vi "RealSense_HelloWorld_Depth_and_Color.vi"() -> ()   [LabVIEW 2023]
doc: "Simple Demo showing how to connect a RealSense Camera to stream COLOR and DEPTH from the stereo camera of a D4xx series camera."
panel:
  out "Output stream format":T1={"width"=1280, "height"=720, "fps"=30, "Profile"=605382696, "ppx"=634.5728, "ppy"=370.69974, "fx"=952.6064, "fy"=952.6064, "model"=4}
  in  "Color Presets":T2(ring)=enum."D435"
  in  "Depth Presets":T3(ring)=enum."Original"
  in  "laser on/off":bool=TRUE
  in  "autoexposure":bool=TRUE
  in  "Laser power, mW":sgl=150.0
  in  "Gain(16-248)":sgl=64.0
  in  "Exposure,us":sgl=156.0
  out "Depth map":sgl[][](graph)
  out "RGB image":picture
  out "iteration":i32=22
  in  "stop":bool=TRUE
  out "release frame error":string="No Error"
  out "Capture1 Error":string="No Error"
  out "Config error":string="No Error\rNo Error"
  out "init results":T4={"camera name"="Intel RealSense 415", "camera S/N"="725112060291", "F/W"="05.08.08.00", "Sensor name"="Stereo Module", "api_version"=20801, "rscontext"=606847696, "device_list"=597043920, "device count"=2, "Dev out"=606875504, "sensor_list"=605604656, "sensor count"=2, "Sensor out"=601640400}
  out "init error":string="No Error\rNo Error\rNo Error\rNo Error\rNo Error\rNo Error\rNo Error\rNo Error\rNo Error\rNo Error\rNo Error"
  out "Close Error":string="No Error\rNo Error\rNo Error\rNo Error"
  out "Start Error":string="No Error\rNo Error\rNo Error"
  out "Capture2 error":string="No Error"
  in  "Select Resolution":u16(ring)=15 items=["424 x 240 @6fps", "424 x 240 @15fps", "424 x 240 @30fps", "424 x 240 @60fps", "424 x 240 @90fps", "480 x 270 @6fps", "480 x 270 @15fps", "480 x 270 @30fps", "480 x 270 @60fps", "480 x 270 @90fps", "640 x 360 @6fps", "640 x 360 @15fps", "640 x 360 @30fps", "640 x 360 @60fps", "640 x 360 @90fps", "640 x 480 @6fps", "640 x 480 @15fps", "640 x 480 @30fps", "640 x 480 @60fps", "640 x 480 @90fps", "848 x 480 @6fps", "848 x 480 @15fps", "848 x 480 @30fps", "848 x 480 @60fps", "848 x 480 @90fps", "1280 x 720 @6fps", "1280 x 720 @15fps", "1280 x 720 @30fps"]
  # "RealSense Hello World: Color + Depth"
  # "This demo shows how to connect a RealSense D4xx Stereo Depth Camera, and stream the COLOR (left) and a DEPTH MAP."
  # "COLOR"
  # "DEPTH MAP"
  # "Note; When you change Depth Preset you need to stop and restart for the HDAD settings to take effect.\n\nTry the Color preset called \"Remove IR2\". It will remove the laser projector from the RGB 1280x720 image."
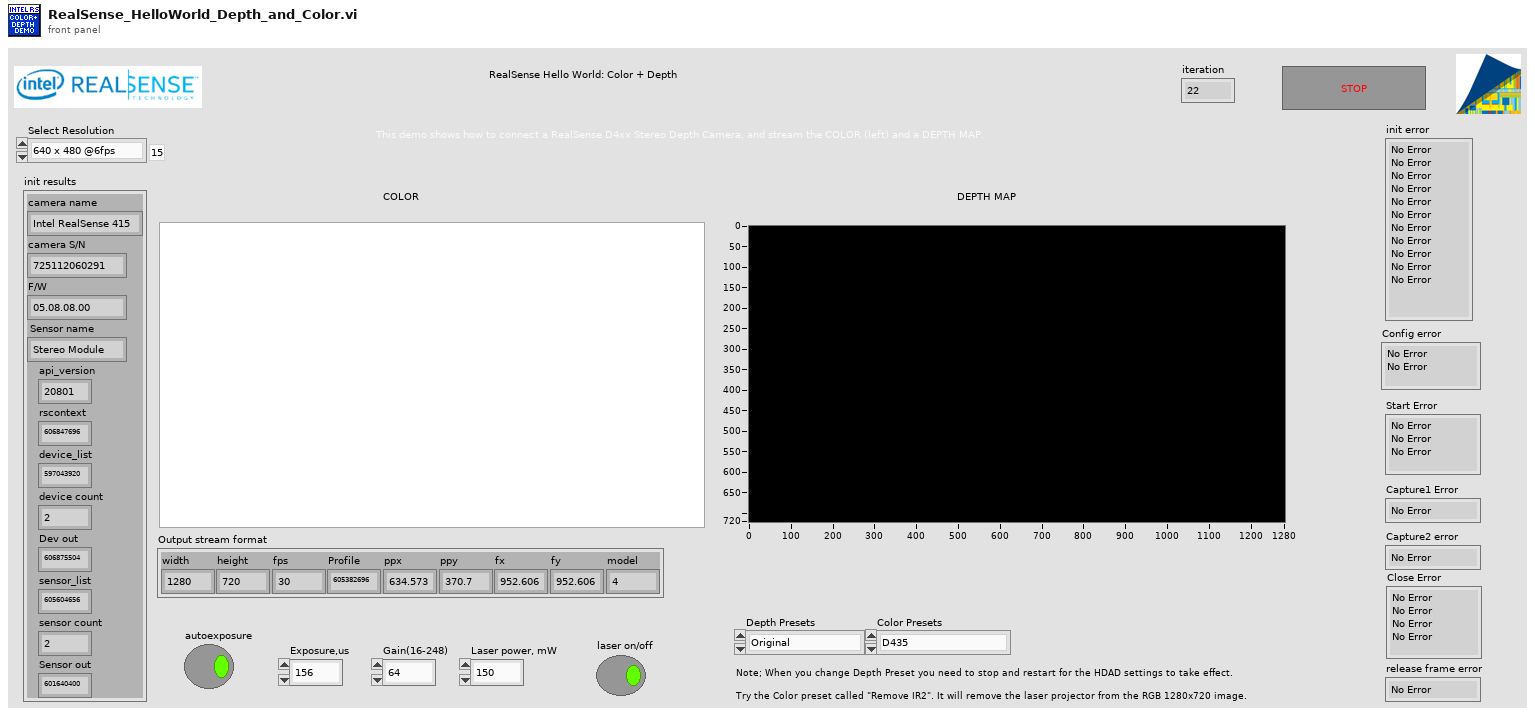
[diagram p1: front panel]
types:
  T1 = cluster{"width":i32, "height":i32, "fps":i32, "Profile":u64, "ppx":sgl, "ppy":sgl, "fx":sgl, "fy":sgl, "model":u32}
  T2 = enum16{"Custom", "RS400 (DS5p)", "RS400 (DS5p) 2", "RS400 (DS5p) 3", "RS400 (DS5p) 4", "RS400 (DS5p) 5", "RS410 (DS5a)", "RS410 (DS5a) 2", "DS410 (DS5a) 3", "DS410 (DS5a) 4", "DS410+IR", "DS5LR", "DS5LR-2", "DS5LR no pattern", "RS410 Remove IR", "RS410 Remove IR 2", "DS5micro", "D435"}
  T3 = enum16{"Custom", "Original", "New Depth 1", "New Depth 2", "Depth Active 1", "Active 3D Scan", "Active Short A", "Active Short C", "Face", "Face2", "Best Box", "High Density", "Medium Density", "High Accuracy", "Hand", "Short Range", "Flat wall", "Load .JSON", "Load .JSON2"}
  T4 = cluster{"camera name":string, "camera S/N":string, "F/W":string, "Sensor name":string, "api_version":i32, "rscontext":u64, "device_list":u64, "device count":i32, "Dev out":u64, "sensor_list":u64, "sensor count":i32, "Sensor out":u64}
  T5 = enum16{"Depth", "Color (ext.)", "Color (left) ", "IR Left", "IR Right", "IR Left (Y16)", "IR Right (Y16)"}
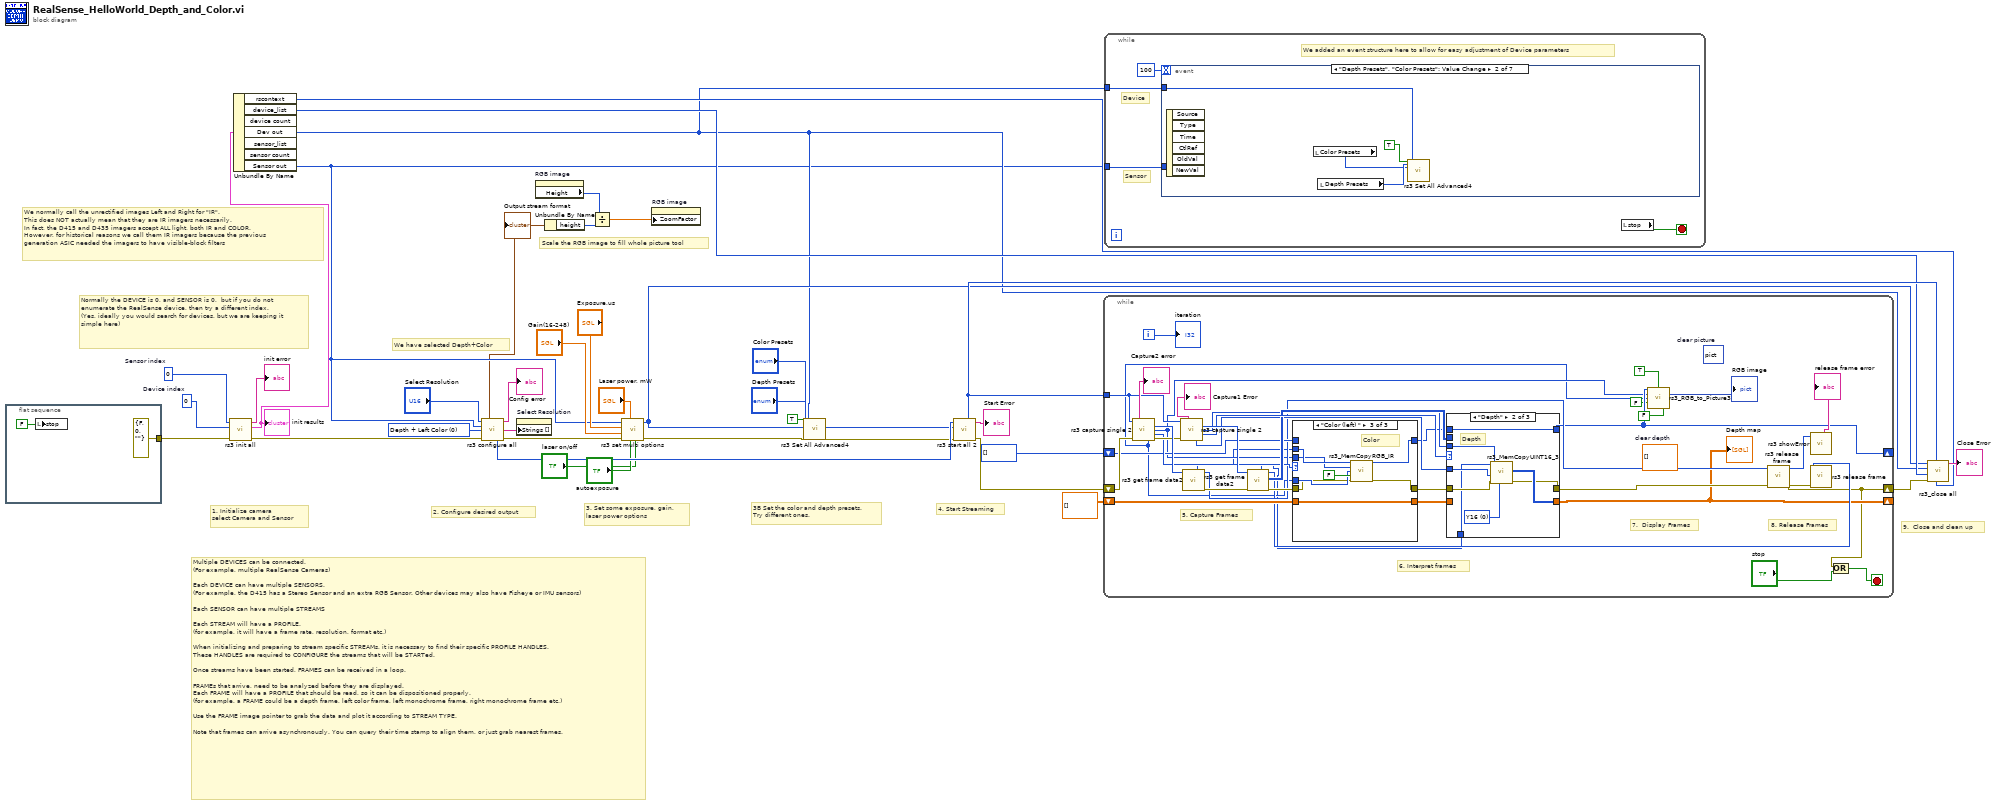
[diagram p0: block diagram]
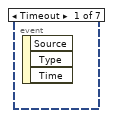
[diagram p2: hidden frame]
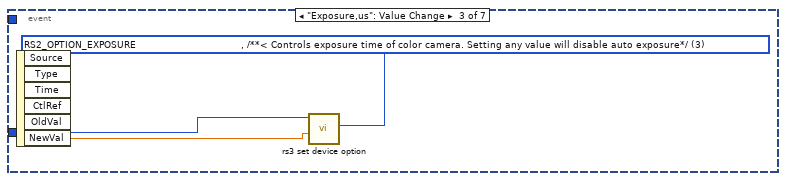
[diagram p3: hidden frame]
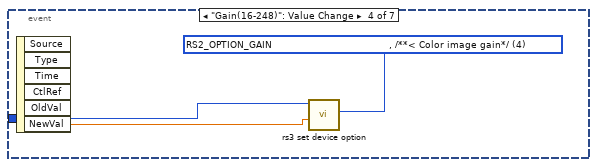
[diagram p4: hidden frame]
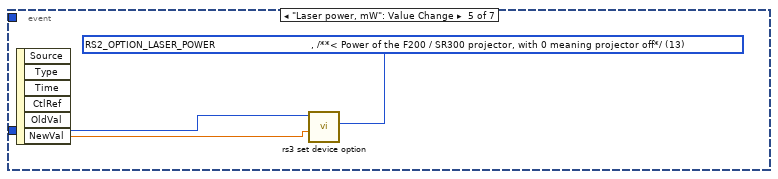
[diagram p5: hidden frame]
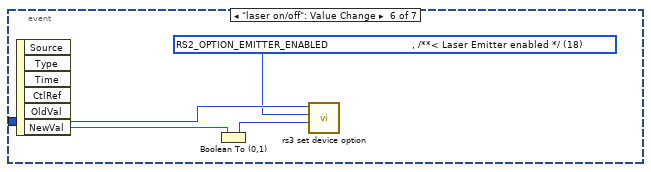
[diagram p6: hidden frame]
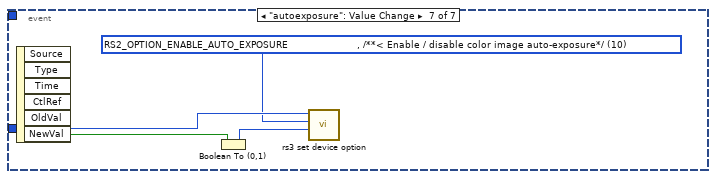
[diagram p7: hidden frame]
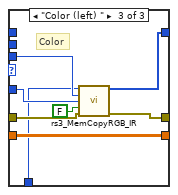
[diagram p9: hidden frame]
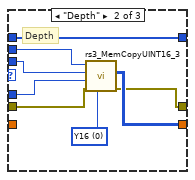
[diagram p11: hidden frame]
diagram:
  w38 = 0  # Device index
  w37 = 0  # Sensor index
  w21 = u16 0 items=["Depth + Left Color", "Unrectified L + R", "Rectified L + R"] ("Stream selection")
  # "Scale the RGB image to fill whole picture tool"
  # "3B Set the color and depth presets.\nTry different ones."
  # "We normally call the unrectified images Left and Right for \"IR\". \nThis does NOT actually mean that they are IR imagers necessarily. \nIn fact, the D415 and D435 imagers accept ALL light, both IR and COLOR.\nHowever, for historical reasons we call them IR imagers because the previous generation ASIC needed the imagers to have visible-block filters"
  # "We have selected Depth+Color"
  # "Normally the DEVICE is 0, and SENSOR is 0,  but if you do not enumerate the RealSense device, then try a different index.\n(Yes, ideally you would search for devices, but we are keeping it simple here)"
  # "Multiple DEVICES can be connected. \n(For example, multiple RealSense Cameras)\n\nEach DEVICE can have multiple SENSORS. \n(For example, the D415 has a Stereo Sensor and an extra RGB Sensor. Other devices may also have Fisheye or IMU sensors) \n\nEach SENSOR can have multiple STREAMS\n\nEach STREAM will have a PROFILE. \n(for example, it will have a frame rate, resolution, format etc.)\n\nWhen initializing and preparing to stream specific STREAMs, it is necessary to find their specific PROFILE HANDLES.\nThese HANDLES are required to CONFIGURE the streams that will be STARTed. \n\nOnce streams have been started, FRAMES can be received in a loop. \n \nFRAMEs that arrive, need to be analyzed before they are displayed. \nEach FRAME will have a PROFILE that should be read, so it can be dispositioned properly.\n(for example, a FRAME could be a depth frame, left color frame, left monochrome frame, right monochrome frame etc.)\n\nUse the FRAME image pointer to grab the data and plot it according to STREAM TYPE.\n\nNote that frames can arrive asynchronously. You can query their time stamp to align them, or just grab nearest frames."
  # "9.  Close and clean up"
  # "4. Start Streaming"
  # "3. Set some exposure, gain, \nlaser power options"
  # "2. Configure desired output"
  # "1. Initialize camera\nselect Camera and Sensor"
  n1 = flat-sequence {
    tunnel: [errorcluster {"status"=FALSE, "code"=0, "source"=""} ("error in")] -> w22
    frame #0 {
      n2 = local write "stop"(FALSE ("stop")) -> ()
    }
  }
  n3 = call "rs3 init all.vi"("error in"=w22, "Select Device"=w38, "Select Sensor"=w37) -> ("error out"=w36:errorcluster, "init results"=w29:T4, "init error"=→"init error":string)  [unwired: 2 in, 4 out]
  "init results" <- w29
  n4 = Unbundle By Name(w29) -> ("rscontext"=w27:u64, "device_list"=w28:u64, "Dev out"=w7:u64, "Sensor out"=w6:u64)  [unwired: 3 out]
  n5 = call "rs3 configure all.vi"("Select Resolution"="Select Resolution", "Sensor in"=w6, "Stream selection"=w21, "error in (no error)"=w36) -> ("Output stream L"=w4:T1, "config error"=→"Config error":string, "Output stream"=w23:string[], "Stream Profile Handles"=w35:u64[], "error out"=w20:errorcluster)  [unwired: 2 in, 5 out]
  "Output stream format" <- w4
  n6 = property on="Select Resolution" class="Ring (strict)"("Strings []"=w23) -> ()  [unwired: 2 in, 2 out]
  n7 = property on="RGB image" class="Pict"() -> ("Height"=w1:u32)  [unwired: 2 in, 2 out]
  n8 = Unbundle By Name(w4) -> ("height"=w2:i32)
  n9 = Divide(x=w1, y=w2) -> (x/y=w3:dbl)
  n10 = call "rs3 set multi options.vi"("laser on/off"="laser on/off", "autoexposure"="autoexposure", "Laser power, mW (0-360)"="Laser power, mW", "error in (no error)"=w20, "Gain(16-248)"="Gain(16-248)", "Exposure, us"="Exposure,us", "Sensor in"=w6) -> ("error out"=w12:errorcluster, "Sensor out"=w19:u64)  [unwired: 2 in, 1 out]
  n11 = property on="RGB image" class="Pict"("ZoomFactor"=w3) -> ()  [unwired: 2 in, 2 out]
  n12 = call "rs3 Set All Advanced4.vi"("Set Color Corr"=TRUE, "Depth Presets"="Depth Presets", "Color Presets"="Color Presets", "error in (no error)"=w12, "device in"=w7) -> ("error out"=w11:errorcluster)  [unwired: 20 in, 2 out]
  n13 = call "rs3 start all 2.vi"("error in (no error)"=w11, "Sensor in"=w19, "Stream profile array"=w35) -> ("error out"=w24:errorcluster, "Config Error"=→"Start Error":string, "queue out"=w34:u64)  [unwired: 5 in, 1 out]
  n14 = while {
    tunnel: w34 -> [w71]
    shift-right: [w46] -> _
    shift-left: sgl[][] [] ("2D Array Output") -> [w59]
    shift-right: [w53] -> _
    shift-left: u8[] [] ("Output Array") -> [w57]
    shift-right: [w41] -> w33
    shift-left: w24 -> [w79]
    i -> [w78]
    stop <- w42 stop-if-true
    (unwired) picture bytes[33]  # clear picture
    (unwired) sgl[][] []  # clear depth
    # "8. Release Frames"
    # "7.  Display Frames"
    # "6. Interpret frames"
    # "5. Capture Frames"
    n15 = call "rs3 capture single 2.vi"("queue in"=w71, "error in (no error)"=w79) -> ("Capture Error"=→"Capture2 error":string, "frame out"=w77:u64, "width"=w51:i32, "Stream type"=w60:T5, "height"=w50:i32, "error out"=w72:errorcluster)  [unwired: 3 in, 5 out]
    n16 = call "rs3 capture single 2.vi"("queue in"=w71, "error in (no error)"=w72) -> ("Capture Error"=→"Capture1 Error":string, "frame out"=w69:u64, "width"=w62:i32, "Stream type"=w64:T5, "height"=w61:i32)  [unwired: 3 in, 6 out]
    n17 = call "rs3 get frame data2.vi"("device in"=w77) -> ("error out"=w75:errorcluster, "device out"=w55:u64, "image pointer out"=w45:u64)  [unwired: 6 in, 2 out]
    n18 = call "rs3 get frame data2.vi"("error in (no error)"=w75, "device in"=w69) -> ("error out"=w74:errorcluster, "2D Depth Output"=w63:u16[][], "device out"=w54:u64, "image pointer out"=w44:u64)  [unwired: 5 in, 1 out]
    n19 = case shown="\"Color (left) \"" w60 {
      tunnel: [w101 w106 w113] -> w66
      tunnel: w45 -> [_ w102 w116]
      tunnel: w51 -> [_ w104 w115]
      tunnel: w50 -> [_ w103 w114]
      tunnel: w74 -> [w101 w107 w112]
      tunnel: [w100 w108 w110] -> w58
      tunnel: w59 -> [w100 _ w110]
      tunnel: w57 -> [w99 w105 _]
      tunnel: [w99 w105 w111] -> w56
      frame "Color (ext.)", Default {
      }
      frame "Depth" {
        w109 = u16 0 items=["Y16", "Y8"] ("Image format")
        # "Depth"
        n20 = call "rs3_MemCopyUINT16_3.vi"("Image format"=w109, "error in (no error)"=w107, "Height"=w103, "Width"=w104, "Zimage pointer"=w102) -> ("error out"=w106:errorcluster, "2D Array Output"=w108:u16[][])  [unwired: 5 in]
      }
      frame "Color (left) " {
        # "Color"
        n21 = call "rs3_MemCopyRGB_IR.vi"("Zimage pointer"=w116, "RGB  X, width"=w115, "RGB Y, height"=w114, "Monochrome(T)/Color(F)"=FALSE ("Grey(T)/Color(F)"), "error in (no error)"=w112) -> ("Output Array"=w111:u8[], "error out"=w113:errorcluster)  [unwired: 9 in]
      }
    }
    n22 = case shown="\"Depth\"" w64 {
      tunnel: [w82 w87 w96] -> w65
      tunnel: w63 -> [_ _ _]
      tunnel: w62 -> [_ w84 w95]
      tunnel: w61 -> [_ w85 w94]
      tunnel: w66 -> [w82 w88 w97]
      tunnel: w58 -> [w81 _ w92]
      tunnel: [w81 w89 w92] -> w46
      tunnel: [w80 w90 w93] -> w53
      tunnel: w56 -> [w80 w90 _]
      tunnel: w44 -> [_ w83 w91]
      frame "Color (ext.)", Default {
      }
      frame "Depth" {
        w86 = u16 0 items=["Y16", "Y8"] ("Image format")
        # "Depth"
        n23 = call "rs3_MemCopyUINT16_3.vi"("Image format"=w86, "error in (no error)"=w88, "Height"=w85, "Width"=w84, "Zimage pointer"=w83) -> ("error out"=w87:errorcluster, "2D Array Output"=w89:u16[][])  [unwired: 5 in]
      }
      frame "Color (left) " {
        # "Color"
        n24 = call "rs3_MemCopyRGB_IR.vi"("Zimage pointer"=w91, "RGB  X, width"=w95, "RGB Y, height"=w94, "Monochrome(T)/Color(F)"=FALSE ("Grey(T)/Color(F)"), "error in (no error)"=w97) -> ("Output Array"=w93:u8[], "error out"=w96:errorcluster)  [unwired: 9 in]
      }
    }
    "Depth map" <- w46
    n25 = call "rs3_RGB_to_Picture3.vi"("RGB array"=w53, "Color(T)/Greyscale(F)"=TRUE, "RGB  X, width"=w51, "RGB Y, height"=w50, "AWB"=FALSE, "White Balance"=FALSE) -> ("new picture"=→"RGB image":picture)  [unwired: 8 in, 1 out]
    n26 = call "rs3 release frame.vi"("error in (no error)"=w65, "Device"=w55) -> ("error out"=w76:errorcluster, "Device out"=w68:u32)  [unwired: 7 in, 1 out]
    n27 = call "rs3 showError.vi"("error"=w68) -> ("Error summary"=→"release frame error":string)  [unwired: 6 in, 4 out]
    n28 = call "rs3 release frame.vi"("error in (no error)"=w76, "Device"=w54) -> ("error out"=w41:errorcluster)  [unwired: 7 in, 2 out]
    n29 = Or(x=w41, y="stop") -> (x .or. y?=w42:bool)
    "iteration" <- w78
  }
  n30 = while {
    tunnel: w7 -> [w120]
    tunnel: w6 -> [w119]
    stop <- w121 stop-if-true
    # "Sensor"
    # "Device"
    # "We added an event structure here to allow for easy adjustment of Device parameters"
    n31 = event shown="[1] \"Depth Presets\", \"Color Presets\": Value Change" {
      selector: _ -> [_ _ _ _ _ _ _]
      dyn-events: _ -> [_ _ _ _ _ _ _]
      timeout: 100 -> [_ _ _ _ _ _ _]
      tunnel: w120 -> [_ w122 _ _ _ _ _]
      tunnel: w119 -> [_ _ w128 w131 w134 w138 w142]
      event Timeout {
        n32 = event-data() -> ()  [unwired: 1 in, 3 out]
      }
      event "Depth Presets", "Color Presets": Value Change {
        n33 = event-data() -> ()  [unwired: 1 in, 6 out]
        n34 = local read "Color Presets"() -> (w124:T2)
        n35 = local read "Depth Presets"() -> (w125:T3)
        n36 = call "rs3 Set All Advanced4.vi"("Set Color Corr"=TRUE, "Depth Presets"=w125, "Color Presets"=w124, "device in"=w122) -> ()  [unwired: 21 in, 3 out]
      }
      event "Exposure,us": Value Change {
        w126 = u16 3 items=["    RS2_OPTION_BACKLIGHT_COMPENSATION                     , /**< Enable / disable color backlight compensation*/", "    RS2_OPTION_BRIGHTNESS                                 , /**< Color image brightness*/", "    RS2_OPTION_CONTRAST                                   , /**< Color image contrast*/", "    RS2_OPTION_EXPOSURE                                   , /**< Controls exposure time of color camera. Setting any value will disable auto exposure*/", "    RS2_OPTION_GAIN                                       , /**< Color image gain*/", "    RS2_OPTION_GAMMA                                      , /**< Color image gamma setting*/", "    RS2_OPTION_HUE                                        , /**< Color image hue*/", "    RS2_OPTION_SATURATION                                 , /**< Color image saturation setting*/", "    RS2_OPTION_SHARPNESS                                  , /**< Color image sharpness setting*/", "    RS2_OPTION_WHITE_BALANCE                              , /**< Controls white balance of color image. Setting any value will disable auto white balance*/", "    RS2_OPTION_ENABLE_AUTO_EXPOSURE                       , /**< Enable / disable color image auto-exposure*/", "    RS2_OPTION_ENABLE_AUTO_WHITE_BALANCE                  , /**< Enable / disable color image auto-white-balance*/", "    RS2_OPTION_VISUAL_PRESET                              , /**< Provide access to several recommend sets of option presets for the depth camera */", "    RS2_OPTION_LASER_POWER                                , /**< Power of the F200 / SR300 projector, with 0 meaning projector off*/", "    RS2_OPTION_ACCURACY                                   , /**< Set the number of patterns projected per frame. The higher the accuracy value the more patterns projected. Increasing the number of patterns help to achieve better accuracy. Note that this c", "    RS2_OPTION_MOTION_RANGE                               , /**< Motion vs. Range trade-off, with lower values allowing for better motion sensitivity and higher values allowing for better depth range*/", "    RS2_OPTION_FILTER_OPTION                              , /**< Set the filter to apply to each depth frame. Each one of the filter is optimized per the application requirements*/", "    RS2_OPTION_CONFIDENCE_THRESHOLD                       , /**< The confidence level threshold used by the Depth algorithm pipe to set whether a pixel will get a valid range or will be marked with invalid range*/", "    RS2_OPTION_EMITTER_ENABLED                            , /**< Laser Emitter enabled */", "    RS2_OPTION_FRAMES_QUEUE_SIZE                          , /**< Number of frames the user is allowed to keep per stream. Trying to hold-on to more frames will cause frame-drops.*/", "    RS2_OPTION_TOTAL_FRAME_DROPS                          , /**< Total number of detected frame drops from all streams */", "    RS2_OPTION_AUTO_EXPOSURE_MODE                         , /**< Auto-Exposure modes: Static, Anti-Flicker and Hybrid */", "    RS2_OPTION_POWER_LINE_FREQUENCY                       , /**< Power Line Frequency control for anti-flickering Off/50Hz/60Hz/Auto */", "    RS2_OPTION_ASIC_TEMPERATURE                           , /**< Current Asic Temperature */", "    RS2_OPTION_ERROR_POLLING_ENABLED                      , /**< disable error handling */", "    RS2_OPTION_PROJECTOR_TEMPERATURE                      , /**< Current Projector Temperature */", "    RS2_OPTION_OUTPUT_TRIGGER_ENABLED                     , /**< Enable / disable trigger to be outputed from the camera to any external device on every depth frame */", "    RS2_OPTION_MOTION_MODULE_TEMPERATURE                  , /**< Current Motion-Module Temperature */", "    RS2_OPTION_DEPTH_UNITS                                , /**< Number of meters represented by a single depth unit */", "    RS2_OPTION_ENABLE_MOTION_CORRECTION                   , /**< Enable/Disable automatic correction of the motion data */", "    RS2_OPTION_AUTO_EXPOSURE_PRIORITY                     , /**< Allows sensor to dynamically ajust the frame rate depending on lighting conditions */", "    RS2_OPTION_COUNT                                      , /**< Number of enumeration values. Not a valid input: intended to be used in for-loops. */"] ("RS Option")
        n37 = event-data() -> ("NewVal"=w127:sgl)  [unwired: 1 in, 5 out]
        n38 = call "rs3 set device option.vi"("value"=w127, "RS Option"=w126, "Sensor in"=w128) -> ()  [unwired: 6 in, 3 out]
      }
      event "Gain(16-248)": Value Change {
        w129 = u16 4 items=["    RS2_OPTION_BACKLIGHT_COMPENSATION                     , /**< Enable / disable color backlight compensation*/", "    RS2_OPTION_BRIGHTNESS                                 , /**< Color image brightness*/", "    RS2_OPTION_CONTRAST                                   , /**< Color image contrast*/", "    RS2_OPTION_EXPOSURE                                   , /**< Controls exposure time of color camera. Setting any value will disable auto exposure*/", "    RS2_OPTION_GAIN                                       , /**< Color image gain*/", "    RS2_OPTION_GAMMA                                      , /**< Color image gamma setting*/", "    RS2_OPTION_HUE                                        , /**< Color image hue*/", "    RS2_OPTION_SATURATION                                 , /**< Color image saturation setting*/", "    RS2_OPTION_SHARPNESS                                  , /**< Color image sharpness setting*/", "    RS2_OPTION_WHITE_BALANCE                              , /**< Controls white balance of color image. Setting any value will disable auto white balance*/", "    RS2_OPTION_ENABLE_AUTO_EXPOSURE                       , /**< Enable / disable color image auto-exposure*/", "    RS2_OPTION_ENABLE_AUTO_WHITE_BALANCE                  , /**< Enable / disable color image auto-white-balance*/", "    RS2_OPTION_VISUAL_PRESET                              , /**< Provide access to several recommend sets of option presets for the depth camera */", "    RS2_OPTION_LASER_POWER                                , /**< Power of the F200 / SR300 projector, with 0 meaning projector off*/", "    RS2_OPTION_ACCURACY                                   , /**< Set the number of patterns projected per frame. The higher the accuracy value the more patterns projected. Increasing the number of patterns help to achieve better accuracy. Note that this c", "    RS2_OPTION_MOTION_RANGE                               , /**< Motion vs. Range trade-off, with lower values allowing for better motion sensitivity and higher values allowing for better depth range*/", "    RS2_OPTION_FILTER_OPTION                              , /**< Set the filter to apply to each depth frame. Each one of the filter is optimized per the application requirements*/", "    RS2_OPTION_CONFIDENCE_THRESHOLD                       , /**< The confidence level threshold used by the Depth algorithm pipe to set whether a pixel will get a valid range or will be marked with invalid range*/", "    RS2_OPTION_EMITTER_ENABLED                            , /**< Laser Emitter enabled */", "    RS2_OPTION_FRAMES_QUEUE_SIZE                          , /**< Number of frames the user is allowed to keep per stream. Trying to hold-on to more frames will cause frame-drops.*/", "    RS2_OPTION_TOTAL_FRAME_DROPS                          , /**< Total number of detected frame drops from all streams */", "    RS2_OPTION_AUTO_EXPOSURE_MODE                         , /**< Auto-Exposure modes: Static, Anti-Flicker and Hybrid */", "    RS2_OPTION_POWER_LINE_FREQUENCY                       , /**< Power Line Frequency control for anti-flickering Off/50Hz/60Hz/Auto */", "    RS2_OPTION_ASIC_TEMPERATURE                           , /**< Current Asic Temperature */", "    RS2_OPTION_ERROR_POLLING_ENABLED                      , /**< disable error handling */", "    RS2_OPTION_PROJECTOR_TEMPERATURE                      , /**< Current Projector Temperature */", "    RS2_OPTION_OUTPUT_TRIGGER_ENABLED                     , /**< Enable / disable trigger to be outputed from the camera to any external device on every depth frame */", "    RS2_OPTION_MOTION_MODULE_TEMPERATURE                  , /**< Current Motion-Module Temperature */", "    RS2_OPTION_DEPTH_UNITS                                , /**< Number of meters represented by a single depth unit */", "    RS2_OPTION_ENABLE_MOTION_CORRECTION                   , /**< Enable/Disable automatic correction of the motion data */", "    RS2_OPTION_AUTO_EXPOSURE_PRIORITY                     , /**< Allows sensor to dynamically ajust the frame rate depending on lighting conditions */", "    RS2_OPTION_COUNT                                      , /**< Number of enumeration values. Not a valid input: intended to be used in for-loops. */"] ("RS Option")
        n39 = event-data() -> ("NewVal"=w130:sgl)  [unwired: 1 in, 5 out]
        n40 = call "rs3 set device option.vi"("value"=w130, "RS Option"=w129, "Sensor in"=w131) -> ()  [unwired: 6 in, 3 out]
      }
      event "Laser power, mW": Value Change {
        w132 = u16 13 items=["    RS2_OPTION_BACKLIGHT_COMPENSATION                     , /**< Enable / disable color backlight compensation*/", "    RS2_OPTION_BRIGHTNESS                                 , /**< Color image brightness*/", "    RS2_OPTION_CONTRAST                                   , /**< Color image contrast*/", "    RS2_OPTION_EXPOSURE                                   , /**< Controls exposure time of color camera. Setting any value will disable auto exposure*/", "    RS2_OPTION_GAIN                                       , /**< Color image gain*/", "    RS2_OPTION_GAMMA                                      , /**< Color image gamma setting*/", "    RS2_OPTION_HUE                                        , /**< Color image hue*/", "    RS2_OPTION_SATURATION                                 , /**< Color image saturation setting*/", "    RS2_OPTION_SHARPNESS                                  , /**< Color image sharpness setting*/", "    RS2_OPTION_WHITE_BALANCE                              , /**< Controls white balance of color image. Setting any value will disable auto white balance*/", "    RS2_OPTION_ENABLE_AUTO_EXPOSURE                       , /**< Enable / disable color image auto-exposure*/", "    RS2_OPTION_ENABLE_AUTO_WHITE_BALANCE                  , /**< Enable / disable color image auto-white-balance*/", "    RS2_OPTION_VISUAL_PRESET                              , /**< Provide access to several recommend sets of option presets for the depth camera */", "    RS2_OPTION_LASER_POWER                                , /**< Power of the F200 / SR300 projector, with 0 meaning projector off*/", "    RS2_OPTION_ACCURACY                                   , /**< Set the number of patterns projected per frame. The higher the accuracy value the more patterns projected. Increasing the number of patterns help to achieve better accuracy. Note that this c", "    RS2_OPTION_MOTION_RANGE                               , /**< Motion vs. Range trade-off, with lower values allowing for better motion sensitivity and higher values allowing for better depth range*/", "    RS2_OPTION_FILTER_OPTION                              , /**< Set the filter to apply to each depth frame. Each one of the filter is optimized per the application requirements*/", "    RS2_OPTION_CONFIDENCE_THRESHOLD                       , /**< The confidence level threshold used by the Depth algorithm pipe to set whether a pixel will get a valid range or will be marked with invalid range*/", "    RS2_OPTION_EMITTER_ENABLED                            , /**< Laser Emitter enabled */", "    RS2_OPTION_FRAMES_QUEUE_SIZE                          , /**< Number of frames the user is allowed to keep per stream. Trying to hold-on to more frames will cause frame-drops.*/", "    RS2_OPTION_TOTAL_FRAME_DROPS                          , /**< Total number of detected frame drops from all streams */", "    RS2_OPTION_AUTO_EXPOSURE_MODE                         , /**< Auto-Exposure modes: Static, Anti-Flicker and Hybrid */", "    RS2_OPTION_POWER_LINE_FREQUENCY                       , /**< Power Line Frequency control for anti-flickering Off/50Hz/60Hz/Auto */", "    RS2_OPTION_ASIC_TEMPERATURE                           , /**< Current Asic Temperature */", "    RS2_OPTION_ERROR_POLLING_ENABLED                      , /**< disable error handling */", "    RS2_OPTION_PROJECTOR_TEMPERATURE                      , /**< Current Projector Temperature */", "    RS2_OPTION_OUTPUT_TRIGGER_ENABLED                     , /**< Enable / disable trigger to be outputed from the camera to any external device on every depth frame */", "    RS2_OPTION_MOTION_MODULE_TEMPERATURE                  , /**< Current Motion-Module Temperature */", "    RS2_OPTION_DEPTH_UNITS                                , /**< Number of meters represented by a single depth unit */", "    RS2_OPTION_ENABLE_MOTION_CORRECTION                   , /**< Enable/Disable automatic correction of the motion data */", "    RS2_OPTION_AUTO_EXPOSURE_PRIORITY                     , /**< Allows sensor to dynamically ajust the frame rate depending on lighting conditions */", "    RS2_OPTION_COUNT                                      , /**< Number of enumeration values. Not a valid input: intended to be used in for-loops. */"] ("RS Option")
        n41 = event-data() -> ("NewVal"=w133:sgl)  [unwired: 1 in, 5 out]
        n42 = call "rs3 set device option.vi"("value"=w133, "RS Option"=w132, "Sensor in"=w134) -> ()  [unwired: 6 in, 3 out]
      }
      event "laser on/off": Value Change {
        w137 = u16 18 items=["    RS2_OPTION_BACKLIGHT_COMPENSATION                     , /**< Enable / disable color backlight compensation*/", "    RS2_OPTION_BRIGHTNESS                                 , /**< Color image brightness*/", "    RS2_OPTION_CONTRAST                                   , /**< Color image contrast*/", "    RS2_OPTION_EXPOSURE                                   , /**< Controls exposure time of color camera. Setting any value will disable auto exposure*/", "    RS2_OPTION_GAIN                                       , /**< Color image gain*/", "    RS2_OPTION_GAMMA                                      , /**< Color image gamma setting*/", "    RS2_OPTION_HUE                                        , /**< Color image hue*/", "    RS2_OPTION_SATURATION                                 , /**< Color image saturation setting*/", "    RS2_OPTION_SHARPNESS                                  , /**< Color image sharpness setting*/", "    RS2_OPTION_WHITE_BALANCE                              , /**< Controls white balance of color image. Setting any value will disable auto white balance*/", "    RS2_OPTION_ENABLE_AUTO_EXPOSURE                       , /**< Enable / disable color image auto-exposure*/", "    RS2_OPTION_ENABLE_AUTO_WHITE_BALANCE                  , /**< Enable / disable color image auto-white-balance*/", "    RS2_OPTION_VISUAL_PRESET                              , /**< Provide access to several recommend sets of option presets for the depth camera */", "    RS2_OPTION_LASER_POWER                                , /**< Power of the F200 / SR300 projector, with 0 meaning projector off*/", "    RS2_OPTION_ACCURACY                                   , /**< Set the number of patterns projected per frame. The higher the accuracy value the more patterns projected. Increasing the number of patterns help to achieve better accuracy. Note that this c", "    RS2_OPTION_MOTION_RANGE                               , /**< Motion vs. Range trade-off, with lower values allowing for better motion sensitivity and higher values allowing for better depth range*/", "    RS2_OPTION_FILTER_OPTION                              , /**< Set the filter to apply to each depth frame. Each one of the filter is optimized per the application requirements*/", "    RS2_OPTION_CONFIDENCE_THRESHOLD                       , /**< The confidence level threshold used by the Depth algorithm pipe to set whether a pixel will get a valid range or will be marked with invalid range*/", "    RS2_OPTION_EMITTER_ENABLED                            , /**< Laser Emitter enabled */", "    RS2_OPTION_FRAMES_QUEUE_SIZE                          , /**< Number of frames the user is allowed to keep per stream. Trying to hold-on to more frames will cause frame-drops.*/", "    RS2_OPTION_TOTAL_FRAME_DROPS                          , /**< Total number of detected frame drops from all streams */", "    RS2_OPTION_AUTO_EXPOSURE_MODE                         , /**< Auto-Exposure modes: Static, Anti-Flicker and Hybrid */", "    RS2_OPTION_POWER_LINE_FREQUENCY                       , /**< Power Line Frequency control for anti-flickering Off/50Hz/60Hz/Auto */", "    RS2_OPTION_ASIC_TEMPERATURE                           , /**< Current Asic Temperature */", "    RS2_OPTION_ERROR_POLLING_ENABLED                      , /**< disable error handling */", "    RS2_OPTION_PROJECTOR_TEMPERATURE                      , /**< Current Projector Temperature */", "    RS2_OPTION_OUTPUT_TRIGGER_ENABLED                     , /**< Enable / disable trigger to be outputed from the camera to any external device on every depth frame */", "    RS2_OPTION_MOTION_MODULE_TEMPERATURE                  , /**< Current Motion-Module Temperature */", "    RS2_OPTION_DEPTH_UNITS                                , /**< Number of meters represented by a single depth unit */", "    RS2_OPTION_ENABLE_MOTION_CORRECTION                   , /**< Enable/Disable automatic correction of the motion data */", "    RS2_OPTION_AUTO_EXPOSURE_PRIORITY                     , /**< Allows sensor to dynamically ajust the frame rate depending on lighting conditions */", "    RS2_OPTION_COUNT                                      , /**< Number of enumeration values. Not a valid input: intended to be used in for-loops. */"] ("RS Option")
        n43 = event-data() -> ("NewVal"=w136:bool)  [unwired: 1 in, 5 out]
        n44 = Boolean To (0,1)(Boolean=w136) -> (0, 1=w135:i16)
        n45 = call "rs3 set device option.vi"("value"=w135, "RS Option"=w137, "Sensor in"=w138) -> ()  [unwired: 6 in, 3 out]
      }
      event "autoexposure": Value Change {
        w141 = u16 10 items=["    RS2_OPTION_BACKLIGHT_COMPENSATION                     , /**< Enable / disable color backlight compensation*/", "    RS2_OPTION_BRIGHTNESS                                 , /**< Color image brightness*/", "    RS2_OPTION_CONTRAST                                   , /**< Color image contrast*/", "    RS2_OPTION_EXPOSURE                                   , /**< Controls exposure time of color camera. Setting any value will disable auto exposure*/", "    RS2_OPTION_GAIN                                       , /**< Color image gain*/", "    RS2_OPTION_GAMMA                                      , /**< Color image gamma setting*/", "    RS2_OPTION_HUE                                        , /**< Color image hue*/", "    RS2_OPTION_SATURATION                                 , /**< Color image saturation setting*/", "    RS2_OPTION_SHARPNESS                                  , /**< Color image sharpness setting*/", "    RS2_OPTION_WHITE_BALANCE                              , /**< Controls white balance of color image. Setting any value will disable auto white balance*/", "    RS2_OPTION_ENABLE_AUTO_EXPOSURE                       , /**< Enable / disable color image auto-exposure*/", "    RS2_OPTION_ENABLE_AUTO_WHITE_BALANCE                  , /**< Enable / disable color image auto-white-balance*/", "    RS2_OPTION_VISUAL_PRESET                              , /**< Provide access to several recommend sets of option presets for the depth camera */", "    RS2_OPTION_LASER_POWER                                , /**< Power of the F200 / SR300 projector, with 0 meaning projector off*/", "    RS2_OPTION_ACCURACY                                   , /**< Set the number of patterns projected per frame. The higher the accuracy value the more patterns projected. Increasing the number of patterns help to achieve better accuracy. Note that this c", "    RS2_OPTION_MOTION_RANGE                               , /**< Motion vs. Range trade-off, with lower values allowing for better motion sensitivity and higher values allowing for better depth range*/", "    RS2_OPTION_FILTER_OPTION                              , /**< Set the filter to apply to each depth frame. Each one of the filter is optimized per the application requirements*/", "    RS2_OPTION_CONFIDENCE_THRESHOLD                       , /**< The confidence level threshold used by the Depth algorithm pipe to set whether a pixel will get a valid range or will be marked with invalid range*/", "    RS2_OPTION_EMITTER_ENABLED                            , /**< Laser Emitter enabled */", "    RS2_OPTION_FRAMES_QUEUE_SIZE                          , /**< Number of frames the user is allowed to keep per stream. Trying to hold-on to more frames will cause frame-drops.*/", "    RS2_OPTION_TOTAL_FRAME_DROPS                          , /**< Total number of detected frame drops from all streams */", "    RS2_OPTION_AUTO_EXPOSURE_MODE                         , /**< Auto-Exposure modes: Static, Anti-Flicker and Hybrid */", "    RS2_OPTION_POWER_LINE_FREQUENCY                       , /**< Power Line Frequency control for anti-flickering Off/50Hz/60Hz/Auto */", "    RS2_OPTION_ASIC_TEMPERATURE                           , /**< Current Asic Temperature */", "    RS2_OPTION_ERROR_POLLING_ENABLED                      , /**< disable error handling */", "    RS2_OPTION_PROJECTOR_TEMPERATURE                      , /**< Current Projector Temperature */", "    RS2_OPTION_OUTPUT_TRIGGER_ENABLED                     , /**< Enable / disable trigger to be outputed from the camera to any external device on every depth frame */", "    RS2_OPTION_MOTION_MODULE_TEMPERATURE                  , /**< Current Motion-Module Temperature */", "    RS2_OPTION_DEPTH_UNITS                                , /**< Number of meters represented by a single depth unit */", "    RS2_OPTION_ENABLE_MOTION_CORRECTION                   , /**< Enable/Disable automatic correction of the motion data */", "    RS2_OPTION_AUTO_EXPOSURE_PRIORITY                     , /**< Allows sensor to dynamically ajust the frame rate depending on lighting conditions */", "    RS2_OPTION_COUNT                                      , /**< Number of enumeration values. Not a valid input: intended to be used in for-loops. */"] ("RS Option")
        n46 = event-data() -> ("NewVal"=w140:bool)  [unwired: 1 in, 5 out]
        n47 = Boolean To (0,1)(Boolean=w140) -> (0, 1=w139:i16)
        n48 = call "rs3 set device option.vi"("value"=w139, "RS Option"=w141, "Sensor in"=w142) -> ()  [unwired: 6 in, 3 out]
      }
    }
    n49 = local read "stop"() -> (w121:bool)
  }
  n50 = call "rs3_close all.vi"("rscontext"=w27, "queue in"=w34, "error in (no error)"=w33, "device_list"=w28, "Dev in"=w7, "Sensor in"=w19) -> ("Close Error"=→"Close Error":string)  [unwired: 4 in, 1 out]
